vi "ELVIS III v1.1 Open AO (Continuous).vi"(8 "error in (no error)":errorcluster, 10 "Channel Names":string[](array[string]), 11 "Resource name":T6 caption="RIO Device") -> (0 "error out":errorcluster, 1 "AO (Continuous) Channels List":T1, 2 "Channel Info":T3, 3 "AO (Continuous) Ref Out":T4 caption="AI Continuous Ref Out")   [LabVIEW 2021]
uses:
  <vilib>/userDefined/High Color/nirio_resource_hc.ctl
  <vilib>/myRIO/Common/Instrument Driver Framework/Utilities/typedefs/myRIO v1.0 Reference.ctl
  <vilib>/myRIO/Common/Instrument Driver Framework/Utilities/typedefs/Generic FPGA Reference.ctl
  <vilib>/myRIO/Common/Instrument Driver Framework/ELVIS III v1.0/AO Continuous/typedefs/AO Continuous Channel Info.ctl
  <vilib>/myRIO/Common/Instrument Driver Framework/ELVIS III v1.0/AO Continuous/typedefs/AO Continuous Channels List.ctl
  <vilib>/myRIO/Common/Instrument Driver Framework/ELVIS III v1.0/AO Continuous/typedefs/ELVIS III v1.0 AO Continuous Channels Enum.ctl
  <vilib>/myRIO/Common/Instrument Driver Framework/myRIO v1.0/AO Continuous/typedefs/AO Continuous Channels Enum.ctl
  <vilib>/myRIO/Common/Instrument Driver Framework/ELVIS III v1.0/AO Continuous/vis/ELVIS III v1.0 Build MUX Configuration AO Continuous.vi
  <vilib>/Utility/VariantDataType/GetNumericInfo.vi
  <vilib>/myRIO/Common/Instrument Driver Framework/ELVIS III v1.0/Resource Manager/vis/ELVIS III v1.0 Reserve Channel List.vi
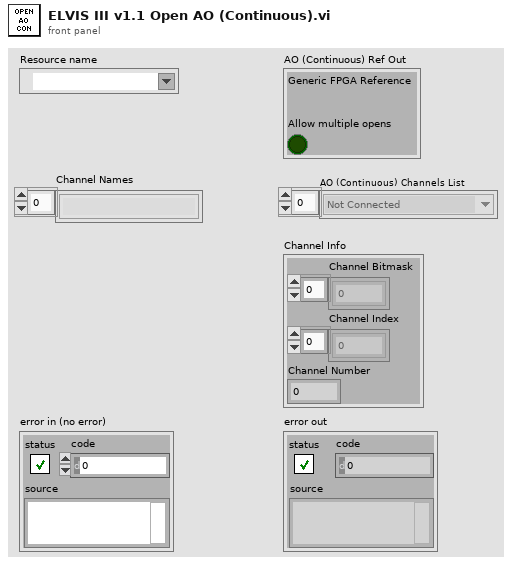
[diagram p1: front panel]
types:
  T1 = typedef "AO Continuous Channels List.ctl" = T2[]
  T2 = typedef "ELVIS III v1.0 AO Continuous Channels Enum.ctl" = enum16{"Not Connected", "A/AO0 (Continuous)", "A/AO1 (Continuous)", "B/AO0 (Continuous)", "B/AO1 (Continuous)"}
  T3 = typedef "AO Continuous Channel Info.ctl" = cluster{"Channel Bitmask":u8[], "Channel Index":i32[], "Channel Number":u8}
  T4 = typedef "myRIO v1.0 Reference.ctl" = cluster{"Generic FPGA Reference":T5, "Allow multiple opens":bool}
  T5 = typedef "Generic FPGA Reference.ctl" = refnum<k20>
  T6 = typedef "nirio_resource_hc.ctl" = tag
  T7 = typedef "AO Continuous Channels Enum.ctl" = enum16{"Not Connected", "A/AO0 (Continuous)", "A/AO1 (Continuous)", "B/AO0 (Continuous)", "B/AO1 (Continuous)"}
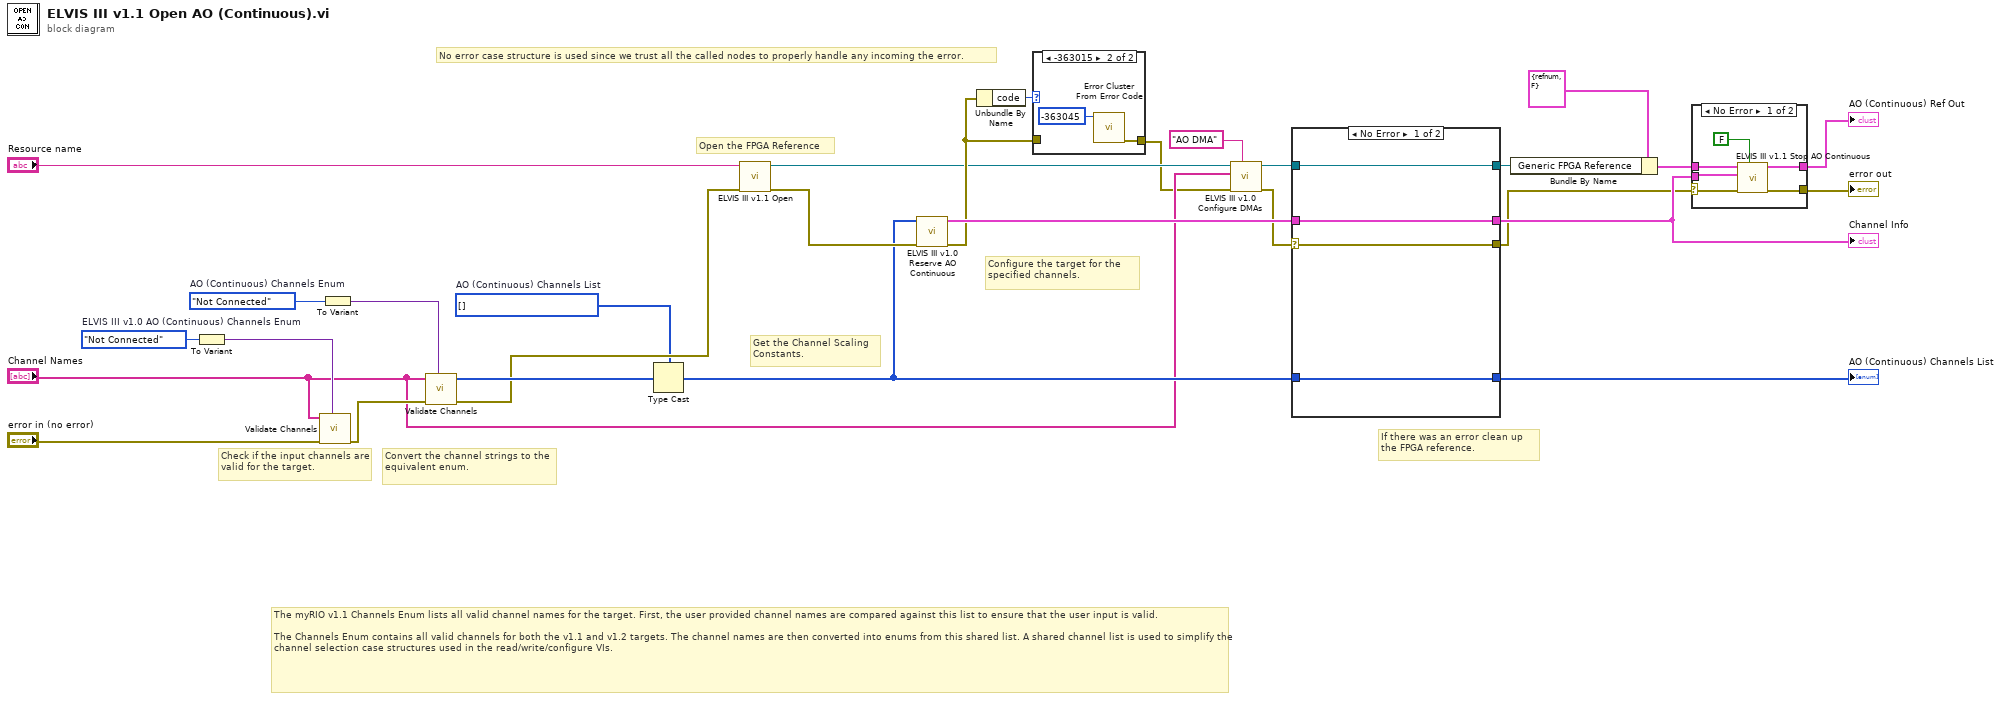
[diagram p0: block diagram]
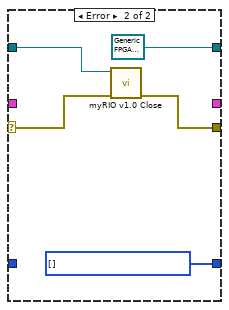
[diagram p4: hidden frame]
diagram:
  w18 = T1 [] items=["Not Connected", "A/AO0 (Continuous)", "A/AO1 (Continuous)", "B/AO0 (Continuous)", "B/AO1 (Continuous)"]  # AO (Continuous) Channels List
  w19 = AO_Continuous_Channels_Enum."Not Connected"  # AO (Continuous) Channels Enum
  w20 = ELVIS_III_v1.0_AO_Continuous_Channels_Enum."Not Connected"  # ELVIS III v1.0 AO (Continuous) Channels Enum
  # "Get the Channel Scaling Constants."
  # "The myRIO v1.1 Channels Enum lists all valid channel names for the target. First, the user provided channel names are compared against this list to ensure that the user input is valid.\n\nThe Channels Enum contains all valid channels for both the v1.1 and v1.2 targets. The channel names are then converted into enums from this shared list. A shared channel list is used to simplify the channel selection case structures used in the read/write/configure VIs."
  # "If there was an error clean up the FPGA reference."
  # "Configure the target for the specified channels."
  # "Open the FPGA Reference"
  # "No error case structure is used since we trust all the called nodes to properly handle any incoming the error."
  # "Convert the channel strings to the equivalent enum."
  # "Check if the input channels are valid for the target."
  n1 = To Variant(anything=w20) -> (Variant=w27:variant)
  n2 = call <vilib>:"Validate Channels.vi"("Channels Enum Variant"=w27, "error in (no error)"="error in (no error)", "Channel Names"="Channel Names") -> ("error out"=w22:errorcluster)  [unwired: 7 in, 1 out]
  n3 = To Variant(anything=w19) -> (Variant=w24:variant)
  n4 = call <vilib>:"Validate Channels.vi"("Channels Enum Variant"=w24, "error in (no error)"=w22, "Channel Names"="Channel Names") -> ("error out"=w21:errorcluster, "Index Array"=w23:u16[])  [unwired: 7 in]
  n5 = Type Cast(type=w18, x=w23) -> (*(type *) &x=w14:T1)
  n6 = call <vilib>:"ELVIS III v1.1 Open.vi"("error in (no error)"=w21, "Resource name"="Resource name") -> ("error out"=w17:errorcluster, "myRIO FPGA Ref Out"=w11:T5)  [unwired: 8 in]
  n7 = call <vilib>:"ELVIS III v1.0 Reserve AO Continuous.vi"("error in (no error)"=w17, "AO (Continuous) Channels List"=w14) -> ("error out"=w12:errorcluster, "Channel Info"=w16:T3)  [unwired: 8 in]
  n8 = Unbundle By Name(w12) -> ("code"=w13:i32)
  n9 = case shown="-363015" w13 {
    tunnel: w12 -> [w30 _]
    tunnel: [w30 w31] -> w8
    frame Default {
    }
    frame -363015 {
      n10 = call <vilib>:"Error Cluster From Error Code.vi"("error code (0)"=-363045) -> ("error out"=w31:errorcluster)  [unwired: 8 in]
    }
  }
  n11 = call <vilib>:"ELVIS III v1.0 Configure DMAs.vi"("DMA Type"="AO DMA", "error in (no error)"=w8, "Channel Names"="Channel Names", "ELVIS III FPGA Ref"=w11) -> ("error out"=w7:errorcluster, "ELVIS III FPGA Ref"=w10:T5)  [unwired: 6 in]
  n12 = case shown="No Error" w7 {
    selector: w7 -> [w35 w41]
    tunnel: w10 -> [w36 w39]
    tunnel: [w36 T5 refnum ("myRIO FPGA Ref Out")] -> w28
    tunnel: [w35 w40] -> w2
    tunnel: [w34 _] -> w3
    tunnel: w16 -> [w34 _]
    tunnel: [w33 w37] -> w15
    tunnel: w14 -> [w33 _]
    frame No Error {
    }
    frame Error {
      w37 = T1 [] items=["Not Connected", "A/AO0 (Continuous)", "A/AO1 (Continuous)", "B/AO0 (Continuous)", "B/AO1 (Continuous)"] ("AO (Continuous) Channels List")
      n13 = call <vilib>:"myRIO v1.0 Close.vi"("error in (no error)"=w41, "myRIO FPGA Ref In"=w39) -> ("error out"=w40:errorcluster)  [unwired: 9 in]
    }
  }
  "Channel Info" <- w3
  "AO (Continuous) Channels List" <- w15
  n14 = Bundle By Name(cluster=T4 {"Generic FPGA Reference"=refnum, "Allow multiple opens"=FALSE} ("myRIO Ref Out"), "Generic FPGA Reference"=w28) -> (w5:T4)
  n15 = case shown="No Error" w2 {
    selector: w2 -> [w43 w48]
    tunnel: w5 -> [w47 w49]
    tunnel: [w46 w49] -> w4
    tunnel: w3 -> [w44 _]
    tunnel: [w42 w48] -> w1
    frame No Error {
      n16 = call <vilib>:"ELVIS III v1.1 Stop AO Continuous.vi"("Wait Until Done?"=FALSE, "error in (no error)"=w43, "Channel Info"=w44, "myRIO Ref In"=w47) -> ("error out"=w42:errorcluster, "myRIO Ref Out"=w46:T4)  [unwired: 6 in]
    }
    frame Error {
    }
  }
  "error out" <- w1
  "AO (Continuous) Ref Out" <- w4
